vi "2d_Array_sortSimplified.vi"(2 "Value":dbl[](array[numeric]), 3 "Time":dbl[](array[numeric])) -> (0 "Dataout":dbl[](array[numeric]), 1 "Timeout":dbl[](array[numeric]))   [LabVIEW 2010]
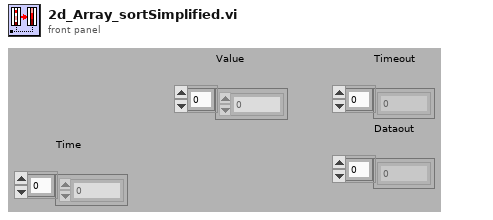
[diagram p1: front panel]
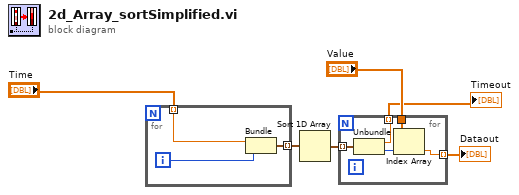
[diagram p0: block diagram]
diagram:
  n1 = for {
    tunnel: "Time" -> [w7] mode=indexing
    tunnel: [w8] -> w4 mode=indexing
    i -> [w9]
    n2 = Bundle(w7, w9) -> (w8:cluster{dbl, i32})  [unwired: 1 out]
  }
  n3 = Sort 1D Array(array=w4) -> (sorted array=w5:cluster{dbl, i32}[])
  n4 = for {
    tunnel: w5 -> [w12] mode=indexing
    tunnel: [w13] -> w1 mode=indexing
    tunnel: "Value" -> [w14]
    tunnel: [w10] -> w2 mode=indexing
    n5 = Unbundle(w12) -> (w10:dbl, w11:i32)
    n6 = Index Array(array=w14, index=w11) -> (element=w13:dbl)
  }
  "Timeout" <- w2
  "Dataout" <- w1
